vi "Write StdOut Log.vi"(8 "error in (no error)":errorcluster, 10 "StdOut Log":refnum<class "Log.lvclass">, 11 "Optimiser Cell in":refnum<class "Optimiser Cell.lvclass">) -> (0 "error out":errorcluster, 3 "Optimiser Cell out":refnum<class "Optimiser Cell.lvclass">)   [LabVIEW 2020, in "CIRCUS_uServices.lvlib" / "Run Utilities.lvlib" / "Optimiser Cell.lvclass"]
uses:
  Optimiser Cell.lvclass
  TALOS/TALOS_PPL.lvlibp/Classes/Log/Log.lvclass
  Optimiser Cell.lvclass/Optimiser Cell.ctl
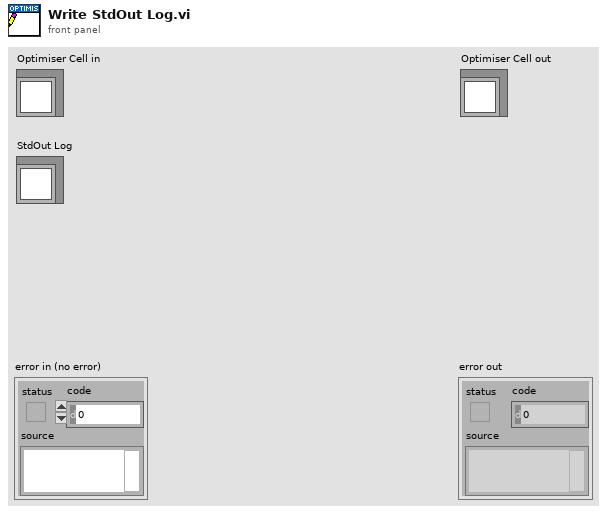
[diagram p1: front panel]
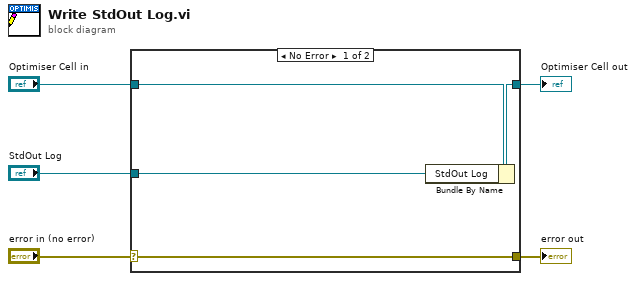
[diagram p0: block diagram]
diagram:
  n1 = case shown="No Error" "error in (no error)" {
    selector: "error in (no error)" -> [w9 w10]
    tunnel: [w9 w10] -> w4
    tunnel: [w7 w11] -> w2
    tunnel: "Optimiser Cell in" -> [w8 w11]
    tunnel: "StdOut Log" -> [w6 _]
    frame No Error {
      n2 = Bundle By Name(cluster=w8, "StdOut Log"=w6) -> (w7:refnum<class "Optimiser Cell.lvclass">)
    }
    frame Error {
    }
  }
  "error out" <- w4
  "Optimiser Cell out" <- w2
